vi "Fault_Logging.vi"(0 "String":string, 5 "Fault Table String Out":string[][](array[string]), 7 "Path":path, 11 "error in (no error)":errorcluster) -> (15 "error out":errorcluster)   [LabVIEW 2021]
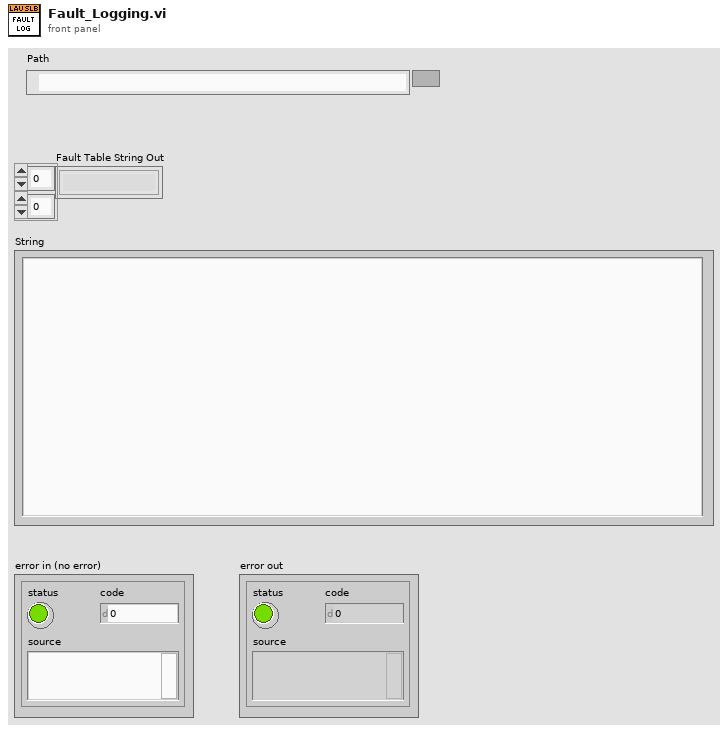
[diagram p1: front panel]
types:
  T1 = enum16{"open", "replace", "create", "open or create", "replace or create", "replace or create with confirmation"}
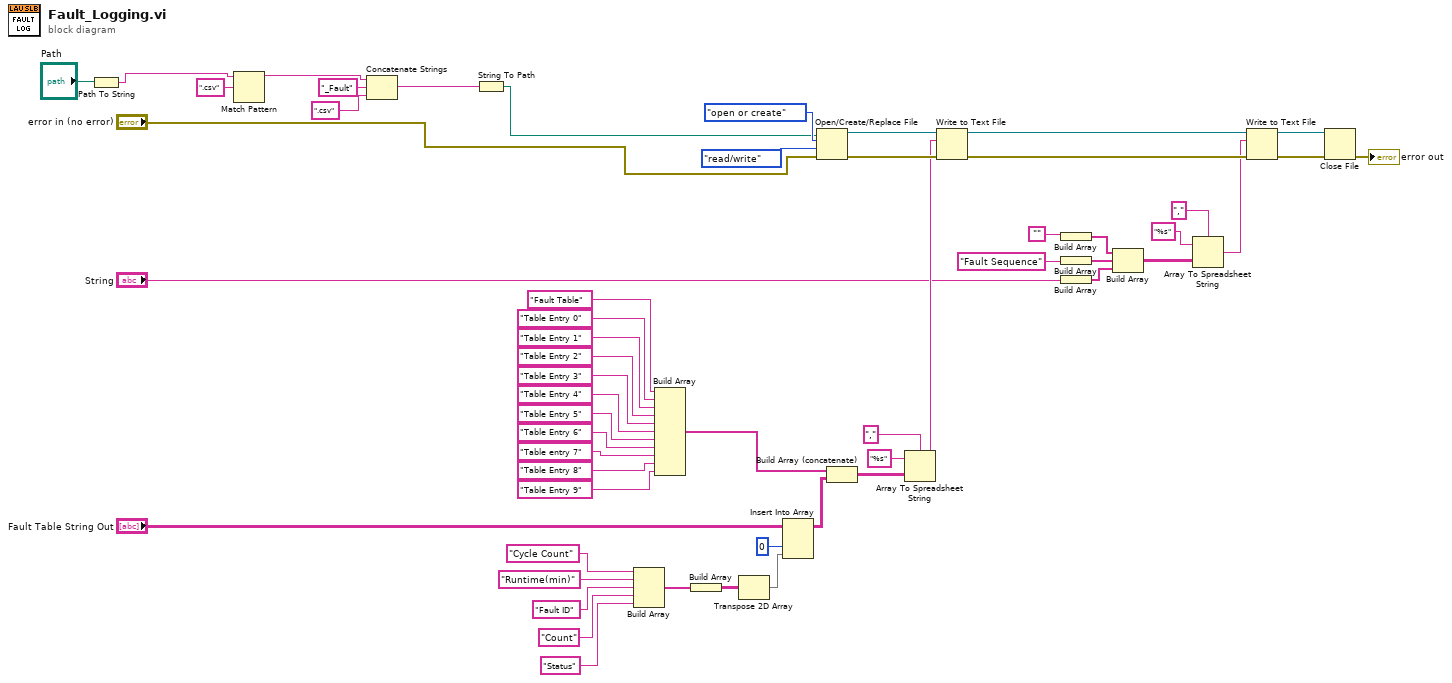
[diagram p0: block diagram]
diagram:
  n1 = Path To String(path="Path") -> (string=w6:string)
  n2 = Match Pattern(string=w6, regular expression=".csv") -> (before substring=w4:string)  [unwired: 1 in, 3 out]
  n3 = Concatenate Strings(w4, "_Fault" ("string"), ".csv" ("string")) -> (w2:string)
  n4 = String To Path(string=w2) -> (path=w1:path)
  n5 = Build Array("Cycle Count" ("delimiter (\\t)"), "Runtime(min)" ("delimiter (\\t)"), "Fault ID" ("delimiter (\\t)"), "Count" ("delimiter (\\t)"), "Status" ("delimiter (\\t)")) -> (w28:string[])
  n6 = Build Array("Fault Table" ("element"), "Table Entry 0" ("delimiter (\\t)"), "Table Entry 1" ("delimiter (\\t)"), "Table Entry 2" ("delimiter (\\t)"), "Table Entry 3" ("delimiter (\\t)"), "Table Entry 4" ("delimiter (\\t)"), "Table Entry 5" ("delimiter (\\t)"), "Table Entry 6" ("delimiter (\\t)"), "Table entry 7" ("delimiter (\\t)"), "Table Entry 8" ("delimiter (\\t)"), "Table Entry 9" ("delimiter (\\t)")) -> (w37:string[])
  n7 = Build Array(w28) -> (w27:string[][])
  n8 = Transpose 2D Array(2D array=w27) -> (transposed array=w25:string[][])
  n9 = Insert Into Array(array="Fault Table String Out", index (col)=0 ("disabled index (col)"), new element=w25) -> (w23:string[][])  [unwired: 1 in]
  n10 = Open/Create/Replace File(file path (use dialog)=w1, error in="error in (no error)", operation (0:open)=T1."open or create", access (0:read/write)=enum16{"read/write", "read-only", "write-only"}."read/write") -> (refnum out=w41:refnum<file>, error out=w40:errorcluster)  [unwired: 2 in, 1 out]
  n11 = Build Array (concatenate)(w37, w23) -> (w36:string[][])
  n12 = Array To Spreadsheet String(delimiter (Tab)=",", array=w36, 3:"%s" ("format string")) -> (spreadsheet string=w35:string)
  n13 = Write to Text File(file (use dialog)=w41, text=w35, error in=w40) -> (refnum out=w22:refnum<file>, error out=w21:errorcluster)  [unwired: 1 in, 1 out]
  n14 = Build Array("") -> (w9:string[])
  n15 = Build Array("Fault Sequence" ("element")) -> (w16:string[])
  n16 = Build Array("String") -> (w15:string[])
  n17 = Build Array(w9, w16, w15) -> (w14:string[][])
  n18 = Array To Spreadsheet String(delimiter (Tab)=",", array=w14, 3:"%s" ("format string")) -> (spreadsheet string=w11:string)
  n19 = Write to Text File(file (use dialog)=w22, text=w11, error in=w21) -> (refnum out=w19:refnum<file>, error out=w20:errorcluster)  [unwired: 1 in, 1 out]
  n20 = Close File(refnum=w19, error in=w20) -> (error out=→"error out":errorcluster)  [unwired: 1 out]
